vi "Write MinWidth.vi"(8 "error in (no error)":errorcluster, 10 "MinWidth":i32=100 min=2 step=1, 11 "GridColumn in":refnum<class "GridColumn.lvclass">) -> (0 "error out":errorcluster, 3 "GridColumn out":refnum<class "GridColumn.lvclass">)   [LabVIEW 2013, in "DataGrid.lvlib" / "GridColumn.lvclass"]
uses:
  GridColumn.lvclass
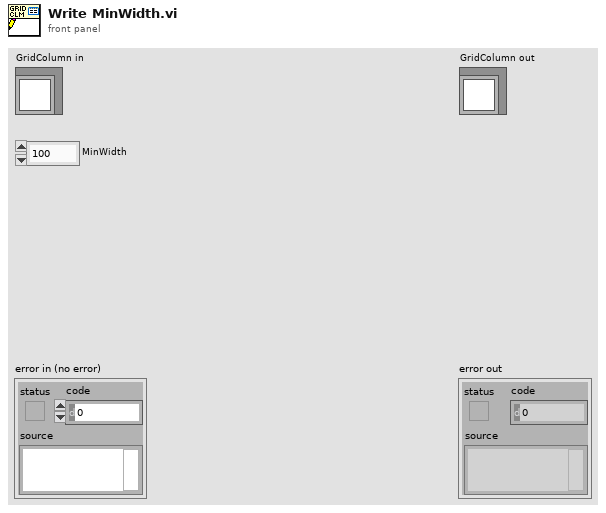
[diagram p1: front panel]
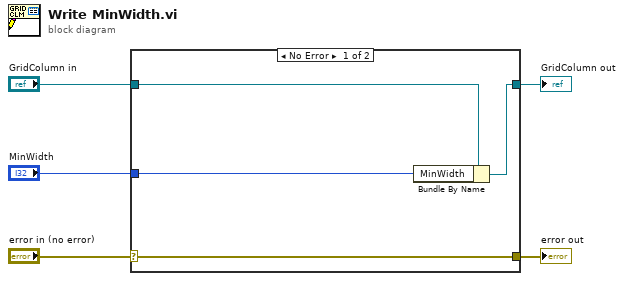
[diagram p0: block diagram]
diagram:
  n1 = case shown="No Error" "error in (no error)" {
    selector: "error in (no error)" -> [w9 w10]
    tunnel: [w9 w10] -> w4
    tunnel: [w7 w11] -> w2
    tunnel: "GridColumn in" -> [w8 w11]
    tunnel: "MinWidth" -> [w6 _]
    frame No Error {
      n2 = Bundle By Name(cluster=w8, "MinWidth"=w6) -> (w7:refnum<class "GridColumn.lvclass">)
    }
    frame Error {
    }
  }
  "error out" <- w4
  "GridColumn out" <- w2
